vi "Pre Enqueue Action.vi"(8 "error in (no error)":errorcluster, 10 "Message Array in":refnum<class "Message.lvclass">[](array[class]), 11 "Msg in":refnum<class "Batch Msg.lvclass">) -> (0 "error out":errorcluster, 2 "Message Array out":refnum<class "Message.lvclass">[](array[class]))   [LabVIEW 2020, in "Sequencer.lvlib" / "Batch Msg.lvclass"]
doc: "Action performed on the message array prior to the enqueue on the Sequencer Core.\n\nThe default implementation does nothing."
uses:
  Batch Msg.lvclass
  PPL/HDH.Actor Framework.Core.Actor.lvlibp/1abvi3w/vi.lib/ActorFramework/Message/Message.lvclass
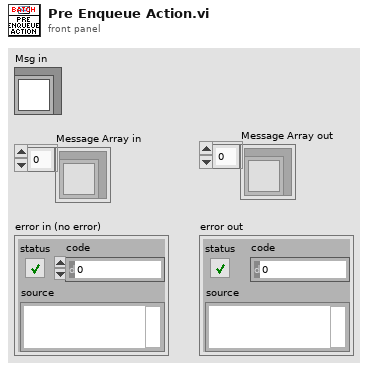
[diagram p1: front panel]
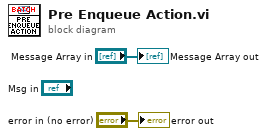
[diagram p0: block diagram]
diagram:
  "Message Array out" <- "Message Array in"
  "error out" <- "error in (no error)"
